vi "GetEverything.vi"() -> ()   [LabVIEW 2019, in "TheConsumer.lvlib" / "TheConsumer.lvclass"]
uses:
  TheConsumer.lvclass
panel:
  out "TheConsumer out":refnum<class "TheConsumer.lvclass">
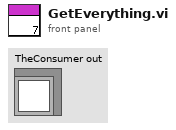
[diagram p1: front panel]
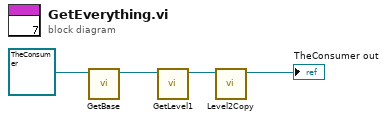
[diagram p0: block diagram]
diagram:
  n1 = call-dynamic "GetBase.vi"("TheConsumer in"=refnum<class "TheConsumer.lvclass"> refnum) -> ("TheConsumer out"=w3:refnum<class "TheConsumer.lvclass">)  [unwired: 8 in, 2 out]
  n2 = call-dynamic "GetLevel1.vi"("TheConsumer in"=w3) -> ("TheConsumer out"=w2:refnum<class "TheConsumer.lvclass">)  [unwired: 8 in, 2 out]
  n3 = call-dynamic "Level2Copy.vi"("TheConsumer in"=w2) -> ("TheConsumer out"=→"TheConsumer out":refnum<class "TheConsumer.lvclass">)  [unwired: 7 in, 3 out]
